vi "Sphere-in-Box test (axis-aligned).vi"(1 "Box":T2, 2 "Sphere":T1) -> (0 "Sphere is inside box":bool)   [LabVIEW 2014]
uses:
  Typedefs/TreeNodeBox.ctl
  Typedefs/Quad.ctl
  Typedefs/Quadplane enum.ctl
  Typedefs/Sphere.ctl
panel:
  # "PN 13/03/2015"
  # "Vertices"
  # "Edges"
  # "Unit normal"
  # "Plane ident."
  # "Vertices"
  # "Edges"
  # "Unit normal"
  # "Plane ident."
  # "Vertices"
  # "Edges"
  # "Unit normal"
  # "Plane ident."
  # "Vertices"
  # "Edges"
  # "Unit normal"
  # "Plane ident."
  # "Vertices"
  # "Edges"
  # "Unit normal"
  # "Plane ident."
  # "Vertices"
  # "Edges"
  # "Unit normal"
  # "Plane ident."
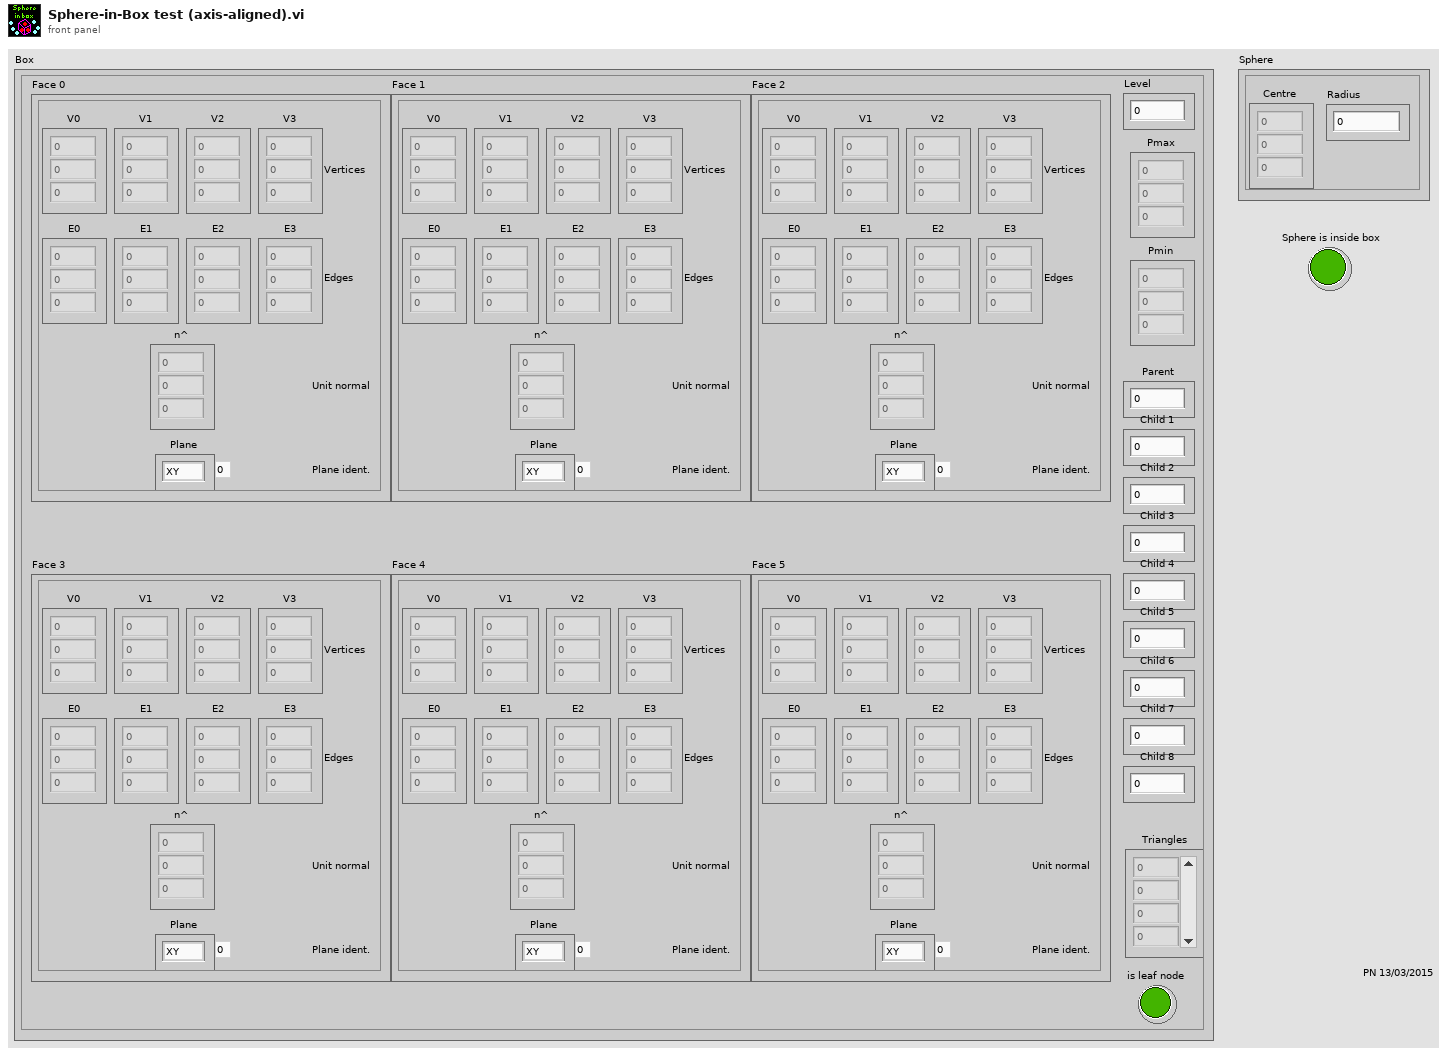
[diagram p1: front panel]
types:
  T1 = typedef "Sphere.ctl" = cluster{"Centre":sgl[], "Radius":sgl}
  T2 = typedef "TreeNodeBox.ctl" = cluster{"Face 0":T3, "Face 1":T3, "Face 2":T3, "Face 3":T3, "Face 4":T3, "Face 5":T3, "Level":i32, "Pmax":sgl[], "Pmin":sgl[], "Parent":i32, "Child 1":i32, "Child 2":i32, "Child 3":i32, "Child 4":i32, "Child 5":i32, "Child 6":i32, "Child 7":i32, "Child 8":i32, "Triangles":i32[], "is leaf node":bool}
  T3 = typedef "Quad.ctl" = cluster{"V0":sgl[], "V1":sgl[], "V2":sgl[], "V3":sgl[], "E0":sgl[], "E1":sgl[], "E2":sgl[], "E3":sgl[], "n^":sgl[], "Plane":T4}
  T4 = typedef "Quadplane enum.ctl" = enum8{"XY", "XZ", "YZ", "-XY", "-XZ", "-YZ"}
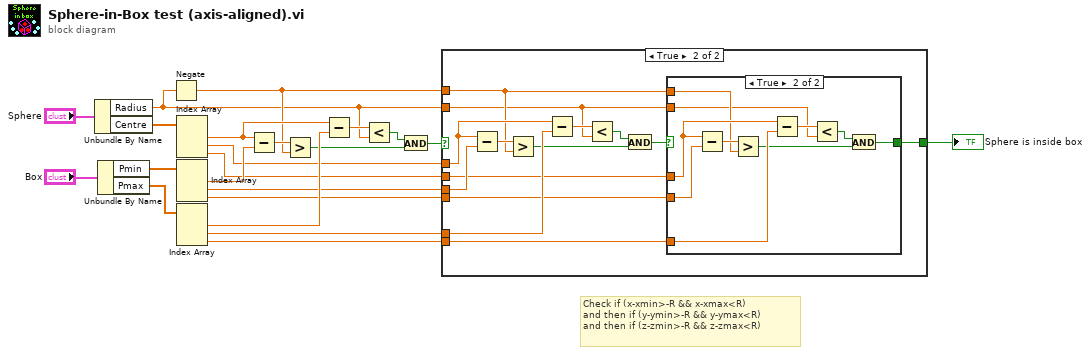
[diagram p0: block diagram]
diagram:
  # "Check if (x-xmin>-R && x-xmax<R)\nand then if (y-ymin>-R && y-ymax<R)\nand then if (z-zmin>-R && z-zmax<R)"
  n1 = Unbundle By Name("Sphere") -> ("Radius"=w8:sgl, "Centre"=w20:sgl[])
  n2 = Unbundle By Name("Box") -> ("Pmin"=w19:sgl[], "Pmax"=w18:sgl[])
  n3 = Negate(x=w8) -> (-x=w10:sgl)
  n4 = Index Array(array=w20) -> (element #1=w15:sgl, element #2=w12:sgl, element #3=w5:sgl)  [unwired: 3 in]
  n5 = Index Array(array=w19) -> (element #1=w17:sgl, element #2=w11:sgl, element #3=w4:sgl)  [unwired: 3 in]
  n6 = Index Array(array=w18) -> (element #1=w14:sgl, element #2=w9:sgl, element #3=w6:sgl)  [unwired: 3 in]
  n7 = Subtract(x=w15, y=w17) -> (x-y=w16:sgl)
  n8 = Greater?(x=w16, y=w10) -> (0:w1:bool)
  n9 = Subtract(x=w15, y=w14) -> (x-y=w13:sgl)
  n10 = Less?(x=w13, y=w8) -> (x < y?=w2:bool)
  n11 = And(x=w2, y=w1) -> (x .and. y?=w3:bool)
  n12 = case shown="True" w3 {
    selector: w3 -> [w23 _]
    tunnel: w12 -> [_ w35]
    tunnel: w11 -> [_ w34]
    tunnel: w10 -> [_ w28]
    tunnel: w9 -> [_ w33]
    tunnel: w8 -> [_ w27]
    tunnel: [w23 w32] -> w7
    tunnel: w6 -> [_ w31]
    tunnel: w5 -> [_ w30]
    tunnel: w4 -> [_ w29]
    frame False {
    }
    frame True {
      n13 = Subtract(x=w35, y=w34) -> (x-y=w36:sgl)
      n14 = Greater?(x=w36, y=w28) -> (0:w24:bool)
      n15 = Subtract(x=w35, y=w33) -> (x-y=w37:sgl)
      n16 = Less?(x=w37, y=w27) -> (x < y?=w26:bool)
      n17 = And(x=w26, y=w24) -> (x .and. y?=w25:bool)
      n18 = case shown="True" w25 {
        selector: w25 -> [w38 _]
        tunnel: [w38 w40] -> w32
        tunnel: w31 -> [_ w46]
        tunnel: w30 -> [_ w45]
        tunnel: w29 -> [_ w44]
        tunnel: w28 -> [_ w43]
        tunnel: w27 -> [_ w42]
        frame False {
        }
        frame True {
          n19 = Subtract(x=w45, y=w44) -> (x-y=w48:sgl)
          n20 = Greater?(x=w48, y=w43) -> (0:w39:bool)
          n21 = Subtract(x=w45, y=w46) -> (x-y=w47:sgl)
          n22 = Less?(x=w47, y=w42) -> (x < y?=w41:bool)
          n23 = And(x=w41, y=w39) -> (x .and. y?=w40:bool)
        }
      }
    }
  }
  "Sphere is inside box" <- w7
